vi "EncenderRIGOLDP832.vi"(8 "error in (no error)":errorcluster, 11 "VISA IN":refnum<visa-resource-name>="FA_Rigol_DP832" caption="VISA resource name") -> (0 "error out":errorcluster, 3 "VISA resource name out":refnum<visa-resource-name>)   [LabVIEW 2019]
uses:
  Rigol DP832/DP832_Control Channels.ctl
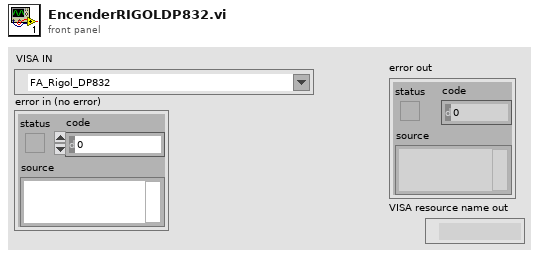
[diagram p1: front panel]
types:
  T1 = typedef "DP832_Control Channels.ctl" = i32
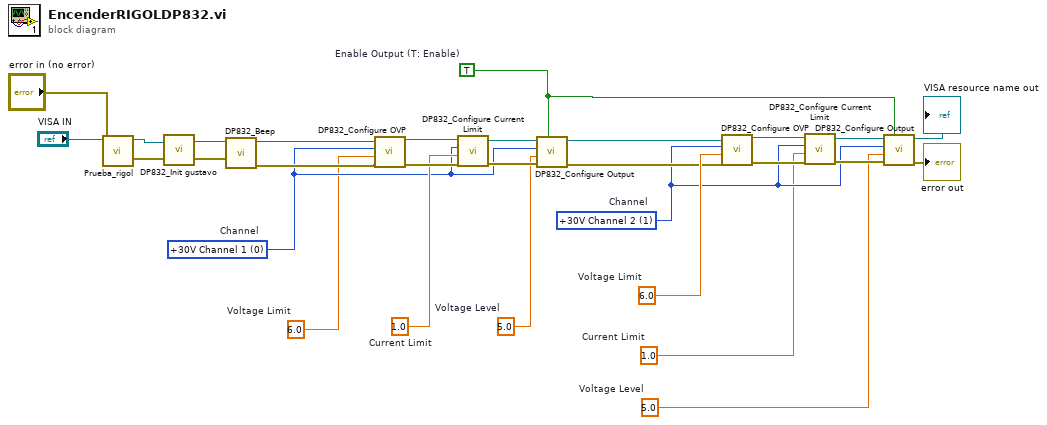
[diagram p0: block diagram]
diagram:
  w5 = 5.0  # Voltage Level
  w6 = 1.0  # Current Limit
  w11 = 6.0  # Voltage Limit
  w7 = T1 1 items=["+30V Channel 1", "+30V Channel 2", "+5V Channel 3"]  # Channel
  w16 = 5.0  # Voltage Level
  w10 = TRUE  # Enable Output (T: Enable)
  w21 = 1.0  # Current Limit
  w17 = 6.0  # Voltage Limit
  w19 = T1 0 items=["+30V Channel 1", "+30V Channel 2", "+5V Channel 3"]  # Channel
  n1 = call "Prueba_rigol.vi"("error in (no error)"="error in (no error)", "VISA IN"="VISA IN") -> ("error out 2"=w28:errorcluster)  [unwired: 8 in, 1 out]
  n2 = call "DP832_Init gustavo.vi"("error in (no error)"=w28, "VISA resource name 2"="VISA IN") -> ("error out"=w27:errorcluster, "VISA resource name"=w26:refnum<visa-resource-name>)
  n3 = call "DP832_Beep.vi"("error in (no error)"=w27, "VISA resource name"=w26) -> ("error out"=w23:errorcluster, "VISA resource name out"=w8:refnum<visa-resource-name>)  [unwired: 8 in]
  n4 = call "DP832_Configure OVP.vi"("error in (no error)"=w23, "Voltage Limit"=w17, "Channel"=w19, "VISA resource name"=w8) -> ("error out"=w22:errorcluster, "VISA resource name out"=w24:refnum<visa-resource-name>)  [unwired: 6 in]
  n5 = call "DP832_Configure Current Limit.vi"("error in (no error)"=w22, "Current Limit"=w21, "Channel"=w19, "VISA resource name"=w24) -> ("error out"=w20:errorcluster, "VISA resource name out"=w18:refnum<visa-resource-name>)  [unwired: 6 in]
  n6 = call "DP832_Configure Output.vi"("Enable Output (T: Enable)"=w10, "error in (no error)"=w20, "Voltage Level"=w16, "Channel"=w19, "VISA resource name"=w18) -> ("error out"=w9:errorcluster, "VISA resource name out"=w4:refnum<visa-resource-name>)  [unwired: 5 in]
  n7 = call "DP832_Configure OVP.vi"("error in (no error)"=w9, "Voltage Limit"=w11, "Channel"=w7, "VISA resource name"=w4) -> ("error out"=w14:errorcluster, "VISA resource name out"=w15:refnum<visa-resource-name>)  [unwired: 6 in]
  n8 = call "DP832_Configure Current Limit.vi"("error in (no error)"=w14, "Current Limit"=w6, "Channel"=w7, "VISA resource name"=w15) -> ("error out"=w13:errorcluster, "VISA resource name out"=w12:refnum<visa-resource-name>)  [unwired: 6 in]
  n9 = call "DP832_Configure Output.vi"("Enable Output (T: Enable)"=w10, "error in (no error)"=w13, "Voltage Level"=w5, "Channel"=w7, "VISA resource name"=w12) -> ("error out"=→"error out":errorcluster, "VISA resource name out"=→"VISA resource name out":refnum<visa-resource-name>)  [unwired: 5 in]
